vi "PiReplaceCodes.vi"(8 "Conv String in":string, 11 "String in":string) -> (0 "String out":string, 3 "Conv String out":string)   [LabVIEW 2019]
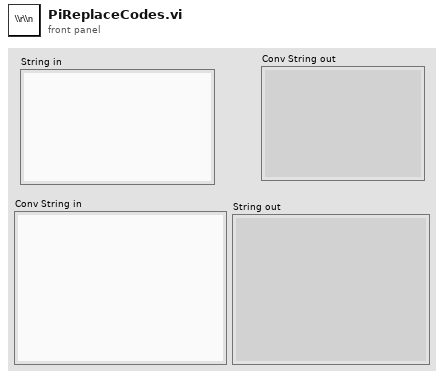
[diagram p1: front panel]
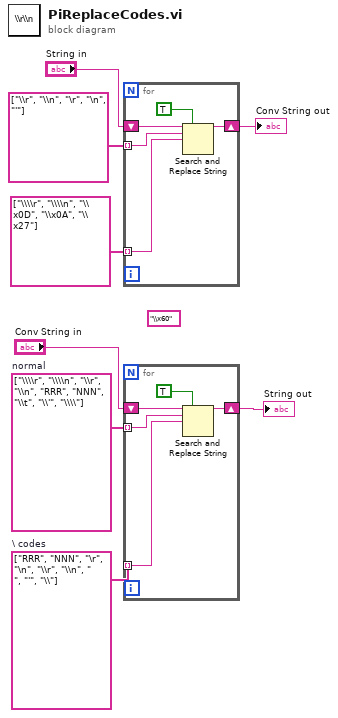
[diagram p0: block diagram]
diagram:
  (unwired) "\\x60"
  w7 = string[] ["\\\\r", "\\\\n", "\\r", "\\n", "RRR", "NNN", "\\t", "\\'", "\\\\"]  # normal
  w6 = string[] ["RRR", "NNN", "\r", "\n", "\\r", "\\n", "     ", "'", "\\"]  # \ codes
  n1 = for {
    shift-right: [w11] -> w2
    shift-left: "String in" -> [w13]
    tunnel: string[] ["\\r", "\\n", "\r", "\n", "'"] -> [w10] mode=indexing
    tunnel: string[] ["\\\\r", "\\\\n", "\\x0D", "\\x0A", "\\x27"] -> [w9] mode=indexing
    n2 = Search and Replace String(replace all?=TRUE ("replace all? (F)"), input string=w13, search string=w10, replace string=w9) -> (result string=w11:string)  [unwired: 4 in, 3 out]
  }
  "Conv String out" <- w2
  n3 = for {
    shift-right: [w16] -> w1
    shift-left: "Conv String in" -> [w17]
    tunnel: w7 -> [w15] mode=indexing
    tunnel: w6 -> [w14] mode=indexing
    n4 = Search and Replace String(replace all?=TRUE ("replace all? (F)"), input string=w17, search string=w15, replace string=w14) -> (result string=w16:string)  [unwired: 4 in, 3 out]
  }
  "String out" <- w1
